vi "GetFileVersion_DotNet.vi"(8 "error in (no error)":errorcluster, 11 "Exe Path":path) -> (0 "error out":errorcluster, 1 "FileVersion":string, 2 "File Info Out":T1, 3 "Exe Path Out":path)   [LabVIEW 2012]
doc: "This VI can obtain information about an existing executable, such as its version, product name, and so on, or it can be called as a subVI from a VI that will be built into an executable to obtain information about that executable.\n\nTo obtain version information about an existing executable, enter a path to an executable into Exe Path and run the Vi.\n\nCall this VI as a subVI from a VI that you will build into an executable and leave the path input unwired to obtain the version information about the built executable."
panel:
  # "This VI can obtain information about an\nexisting executable, such as its\nversion, product name, and so on, or it\ncan be called as a subVI from a VI\nthat will be built into an executable to\nobtain information about that\nexecutable.\n\nTo obtain version information about an\nexisting executable, enter a path to an\nexecutable into Exe Path and run the Vi.\n\nCall this VI as a subVI from a VI that\nyou will build into an executable and\nleave the path input unwired to\nobtain the version information about\nthe built executable."
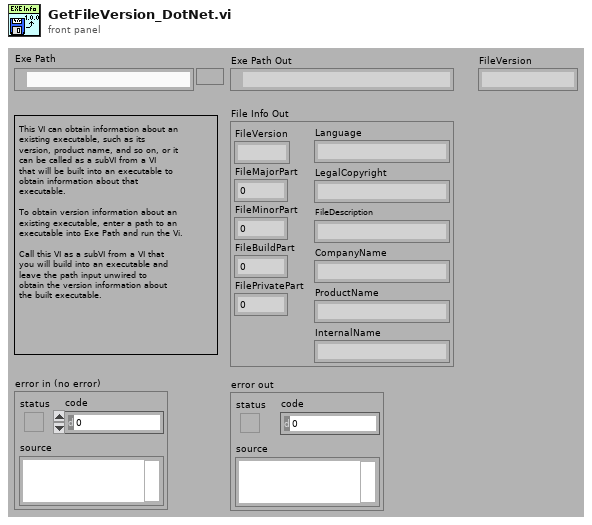
[diagram p1: front panel]
types:
  T1 = cluster{"FileVersion":string, "FileMajorPart":i32, "FileMinorPart":i32, "FileBuildPart":i32, "FilePrivatePart":i32, "Language":string, "LegalCopyright":string, "FileDescription":string, "CompanyName":string, "ProductName":string, "InternalName":string}
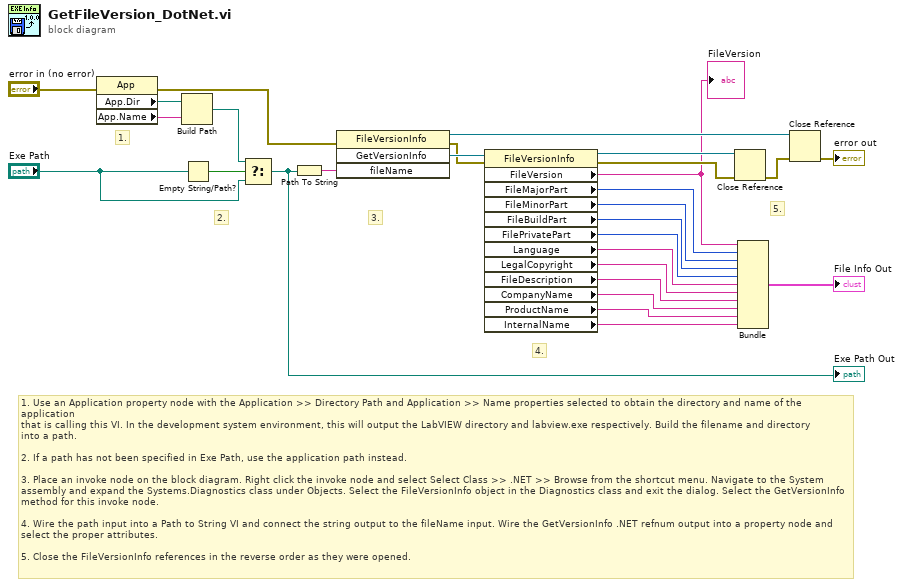
[diagram p0: block diagram]
diagram:
  # "1. Use an Application property node with the Application >> Directory Path and Application >> Name properties selected to obtain the directory and name of the application \nthat is calling this VI. In the development system environment, this will output the LabVIEW directory and labview.exe respectively. Build the filename and directory\ninto a path.\n\n2. If a path has not been specified in Exe Path, use the application path instead.\n\n3. Place an invoke node on the block diagram. Right click the invoke node and select Select Class >> .NET >> Browse from the shortcut menu. Navigate to the System\nassembly and expand the Systems.Diagnostics class under Objects. Select the FileVersionInfo object in the Diagnostics class and exit the dialog. Select the GetVersionInfo\nmethod for this invoke node.\n\n4. Wire the path input into a Path to String VI and connect the string output to the fileName input. Wire the GetVersionInfo .NET refnum output into a property node and\nselect the proper attributes.\n\n5. Close the FileVersionInfo references in the reverse order as they were opened."
  # "5."
  # "4."
  # "1."
  # "3."
  # "2."
  n1 = property class="App"(error in="error in (no error)") -> (error out=w14:errorcluster, "App.Dir"=w23:path, "App.Name"=w22:string)  [unwired: 1 in, 1 out]
  n2 = Build Path(base path=w23, name or relative path=w22) -> (appended path=w19:path)
  n3 = Empty String/Path?(string/path="Exe Path") -> (empty?=w21:bool)
  n4 = Select(t=w19, s=w21, f="Exe Path") -> (s? t:f=w18:path)
  "Exe Path Out" <- w18
  n5 = Path To String(path=w18) -> (string=w26:string)
  n6 = invoke class="FileVersionInfo" method="GetVersionInfo"(error in=w14, "fileName"=w26) -> (reference out=w15:refnum<k24>, error out=w27:errorcluster, "GetVersionInfo"=w28:refnum<k24>)  [unwired: 2 in, 1 out]
  n7 = property class="FileVersionInfo"(reference=w28, error in=w27) -> (reference out=w25:refnum<k24>, error out=w24:errorcluster, "FileVersion"=w12:string, "FileMajorPart"=w11:i32, "FileMinorPart"=w10:i32, "FileBuildPart"=w9:i32, "FilePrivatePart"=w8:i32, "Language"=w7:string, "LegalCopyright"=w6:string, "FileDescription"=w5:string, "CompanyName"=w4:string, "ProductName"=w3:string, "InternalName"=w2:string)
  "FileVersion" <- w12
  n8 = Close Reference(reference=w25, error in (no error)=w24) -> (error out=w16:errorcluster)
  n9 = Bundle("FileVersion"=w12, "FileMajorPart"=w11, "FileMinorPart"=w10, "FileBuildPart"=w9, "FilePrivatePart"=w8, "Language"=w7, "LegalCopyright"=w6, "FileDescription"=w5, "CompanyName"=w4, "ProductName"=w3, "InternalName"=w2) -> (→"File Info Out":T1)  [unwired: 1 in]
  n10 = Close Reference(reference=w15, error in (no error)=w16) -> (error out=→"error out":errorcluster)
